vi "W2Q3.vi"() -> ()   [LabVIEW 2023]
panel:
  out "nPr":dbl
  out "nCr":dbl
  in  "R":dbl
  in  "N":dbl
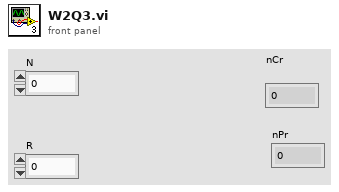
[diagram p1: front panel]
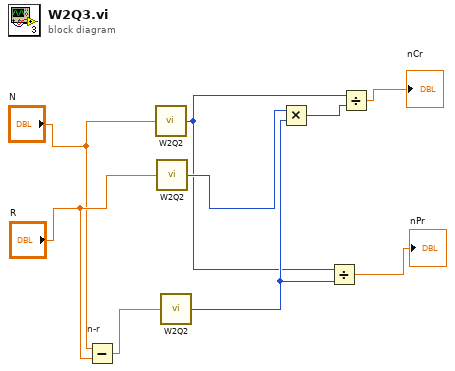
[diagram p0: block diagram]
diagram:
  n1 = Subtract "n-r"(x="N", y="R") -> (x-y=w4:dbl)
  n2 = call "W2Q2.vi"("Numeric 2"="N") -> ("Numeric"=w1:i32)
  n3 = call "W2Q2.vi"("Numeric 2"="R") -> ("Numeric"=w5:i32)
  n4 = call "W2Q2.vi"("Numeric 2"=w4) -> ("Numeric"=w3:i32)
  n5 = Multiply(x=w5, y=w3) -> (x*y=w9:i32)
  n6 = Divide(x=w1, y=w3) -> (x/y=→"nPr":dbl)
  n7 = Divide(x=w1, y=w9) -> (x/y=→"nCr":dbl)
